vi "LIA.GetPublicEventsRegistration.vi"(8 "error in (no error)":errorcluster, 11 "LIA":refnum<class "LIA.lvclass">) -> (0 "error out":errorcluster, 2 "LIA Public Events":refnum<event-registration>, 3 "LIA out":refnum<class "LIA.lvclass">)   [LabVIEW 2017, in "LIA.lvclass"]
doc: "---------------------------------------------------------------\nJKI State Machine Objects™\nhttp://jki.net/state-machine-objects/\nCopyright (C) 2005-2015, JKI <info@jki.net>\nALL RIGHTS RESERVEDJKI State Machine Objects (SMO) 1.0.0.5\nJKI - JKI\nCopyright (c) 2016, JKI"
uses:
  LIA.lvclass
  MeasuringDevice/Typedefs/PublicEvents--Cluster.ctl
  MeasuringDevice/Typedefs/PublicEvents--MeasuringDevice.MeasurementCompleted.ctl
  D:/upwork/Laser Measurement Tool/Laser/project/Subsystems/MeasuringDevice/MeasuringDevice.lvclass
  MeasuringDevice/MeasuringDevice.lvclass
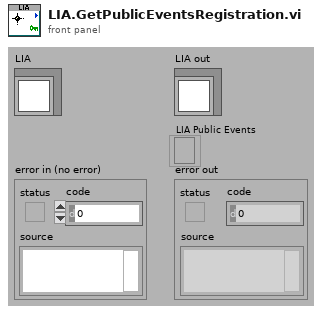
[diagram p1: front panel]
types:
  T1 = typedef "MeasuringDevice.lvclass/PublicEvents--Cluster.ctl" = cluster{"MeasurementCompleted":refnum<user-event>}
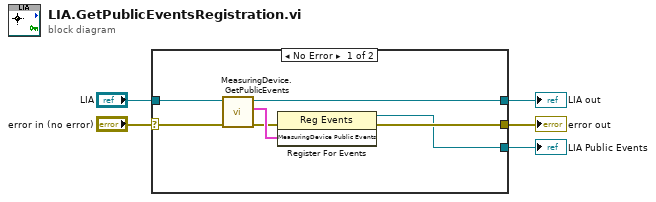
[diagram p0: block diagram]
diagram:
  n1 = case shown="No Error" "error in (no error)" {
    selector: "error in (no error)" -> [w6 w13]
    tunnel: "LIA" -> [w11 w14]
    tunnel: [w9 w13] -> w5
    tunnel: [w10 w14] -> w2
    tunnel: [w8 _] -> w3
    frame No Error {
      n2 = call "MeasuringDevice.GetPublicEvents.vi"("error in (no error)"=w6, "MeasuringDevice"=w11) -> ("error out"=w7:errorcluster, "MeasuringDevice Public Events"=w12:T1, "MeasuringDevice out"=w10:refnum<class "LIA.lvclass">)  [unwired: 7 in]
      n3 = register-events(error in=w7, w12) -> (reference out=w8:refnum<event-registration>, error out=w9:errorcluster)  [unwired: 1 in]
    }
    frame Error {
    }
  }
  "error out" <- w5
  "LIA Public Events" <- w3
  "LIA out" <- w2
